vi "PH_PSDBWriter.get Instance IDs.vi"(1 "PSDB Credentials":T1={"PW"="N/A", "ID"="N/A", "DS"="N/A"}, 3 "Instances":T2(array[cluster]), 5 "error in":errorcluster) -> (16 "Instance IDs":i32[](array[numeric]), 19 "error out":errorcluster)   [LabVIEW 2014, in "PH_PSDBWriter.lvlib"]
uses:
  PH_PSDBWriter.lvlib
  PH_Common/Connection/PH_Connection.PSDB Credentials.ctl
  CSlibraries-extern/psdb_lv/PSDB.lvlib
  PH_Common/PH_Common.lvlib
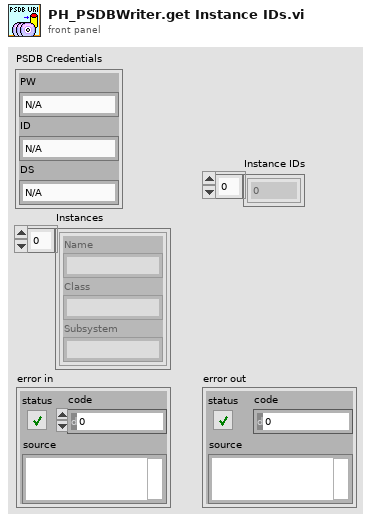
[diagram p1: front panel]
types:
  T1 = typedef "PH_Common.lvlib/PH_Connection.PSDB Credentials.ctl" = cluster{"PW":string, "ID":string, "DS":string}
  T2 = cluster{"Name":string, "Class":string, "Subsystem":string}[]
  T3 = typedef "NI_Database_API.lvlib/Conn ObjectReference.ctl" = refnum<k1>
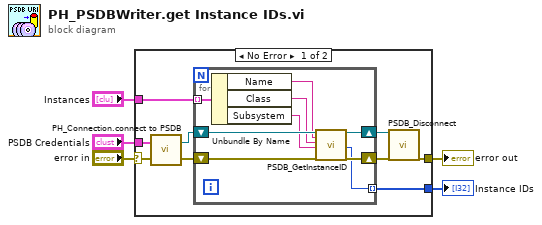
[diagram p0: block diagram]
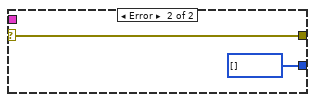
[diagram p2: hidden frame]
diagram:
  n1 = case shown="No Error" "error in" {
    selector: "error in" -> [w7 w25]
    tunnel: [w14 w25] -> w5
    tunnel: [w9 i32[] []] -> w3
    tunnel: "Instances" -> [w8 _]
    tunnel: "PSDB Credentials" -> [w6 _]
    frame No Error {
      n2 = call "PH_Connection.connect to PSDB.vi"("error in"=w7, "PSDB Credentials"=w6) -> ("error out"=w13:errorcluster, "connection reference"=w12:T3)
      n3 = for {
        tunnel: [w19] -> w9 mode=indexing
        tunnel: w8 -> [w18] mode=indexing
        shift-right: [w20] -> w10
        shift-left: w13 -> [w23]
        shift-right: [w21] -> w11
        shift-left: w12 -> [w22]
        n4 = Unbundle By Name(w18) -> ("Name"=w15:string, "Class"=w16:string, "Subsystem"=w17:string)
        n5 = call "PSDB_GetInstanceID.vi"("connection reference"=w22, "Instance"=w15, "Classtype"=w16, "Subsystem"=w17, "error in (no error)"=w23) -> ("connection reference out"=w21:T3, "instance_id"=w19:i32, "error out"=w20:errorcluster)  [unwired: 12 in]
      }
      n6 = call "PSDB_Disconnect.vi"("connection reference"=w11, "error in (no error)"=w10) -> ("error out"=w14:errorcluster)  [unwired: 17 in]
    }
    frame Error {
    }
  }
  "error out" <- w5
  "Instance IDs" <- w3
